vi "HomeMoveTo.vi"(4 "Curr Pos":dbl, 5 "Start Pos":dbl, 6 "Distance from lim to home":dbl, 7 "Axis Name":string, 8 "Which Limit":dbl, 9 "Stage Range":dbl, 10 "Steps/unit":dbl, 11 "Homes?":bool) -> ()   [LabVIEW 2015]
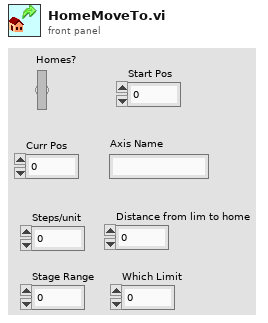
[diagram p1: front panel]
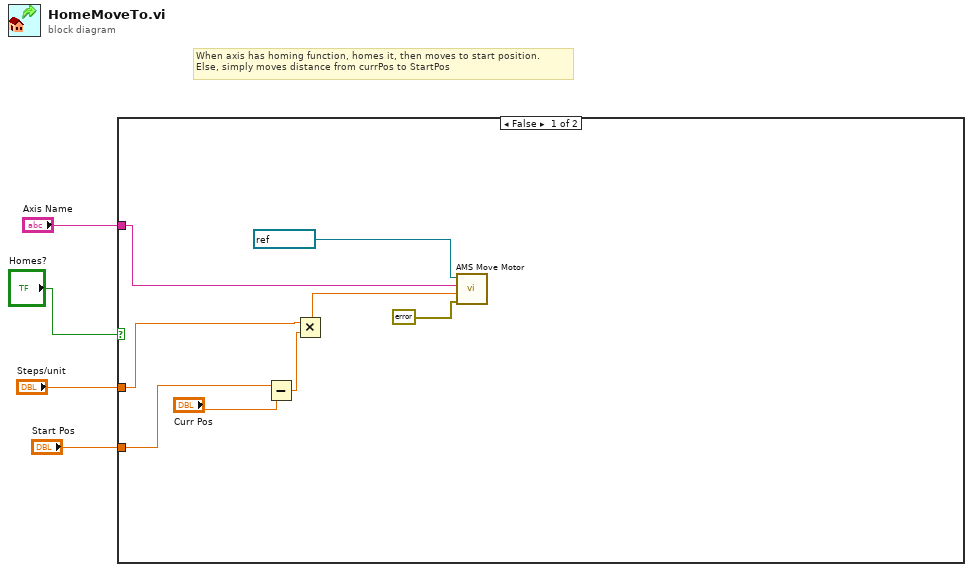
[diagram p0: block diagram]
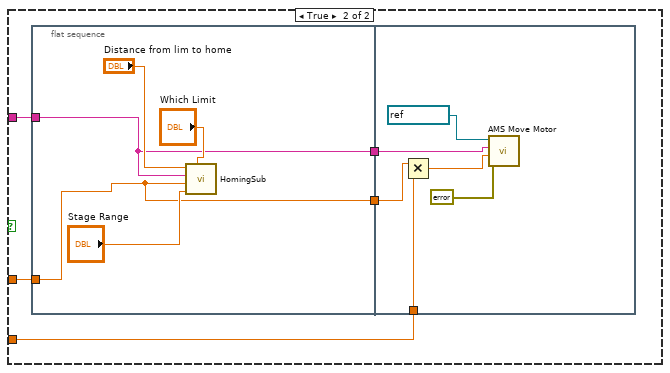
[diagram p2: hidden frame]
diagram:
  # "When axis has homing function, homes it, then moves to start position.\nElse, simply moves distance from currPos to StartPos"
  n1 = case shown="False" "Homes?" {
    tunnel: "Start Pos" -> [w10 w15]
    tunnel: "Steps/unit" -> [w8 w14]
    tunnel: "Axis Name" -> [w11 w13]
    frame False {
      n2 = Subtract(x=w10, y="Curr Pos") -> (x-y=w7:dbl)
      n3 = Multiply(x=w8, y=w7) -> (x*y=w6:dbl)
      n4 = call "AMS Move Motor.vi"("error in"=errorcluster {"status"=FALSE, "code"=0, "source"=""} ("error constant"), "Motor steps"=w6, "Axis Prefix"=w11, "VISA resource name IN"=refnum<visa-resource-name> "COM5") -> ()  [unwired: 6 in, 2 out]
    }
    frame True {
      n5 = flat-sequence {
        tunnel: [w18] -> w17
        tunnel: [w19] -> w16
        tunnel: w14 -> [w19]
        tunnel: w13 -> [w18]
        tunnel: w17 -> [w27]
        tunnel: w16 -> [w25]
        tunnel: w15 -> [w24]
        frame #0 {
          n6 = call "HomingSub.vi"("Which Limit? (0/1)"="Which Limit", "Stage Range"="Stage Range", "Steps/(cm/degree)"=w19, "Controller Name"=w18, "Distance from limit to home (cm/degrees)"="Distance from lim to home") -> ()  [unwired: 6 in, 1 out]
        }
        frame #1 {
          n7 = Multiply(x=w25, y=w24) -> (x*y=w26:dbl)
          n8 = call "AMS Move Motor.vi"("error in"=errorcluster {"status"=FALSE, "code"=0, "source"=""} ("error constant"), "Motor steps"=w26, "Axis Prefix"=w27, "VISA resource name IN"=refnum<visa-resource-name> "COM5") -> ()  [unwired: 6 in, 2 out]
        }
      }
    }
  }
